vi "Query Capabilities (Aperture).vi"(0 "VISA resource name":refnum<visa-resource-name>, 5 "Absolute Maximums (T)":bool=TRUE, 11 "error in (no error)":errorcluster) -> (4 "VISA resource name out":refnum<visa-resource-name>, 6 "Aperture Min (s)":dbl, 8 "Aperture Max (s)":dbl, 15 "error out":errorcluster)   [LabVIEW 2012, in "NH Research Regenerative Test Series.lvlib"]
doc: "Returns the aperture capabilities of the module in seconds."
uses:
  <instrlib>/NH Research Regenerative Test Series/NH Research Regenerative Test Series.lvlib
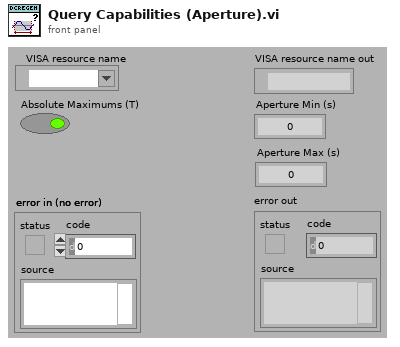
[diagram p1: front panel]
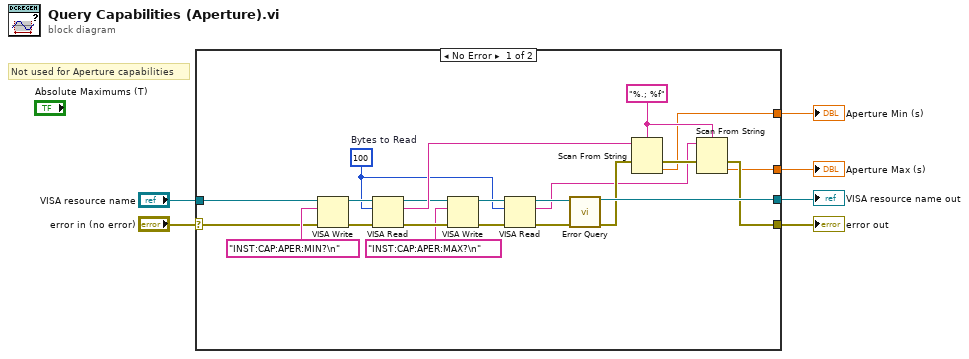
[diagram p0: block diagram]
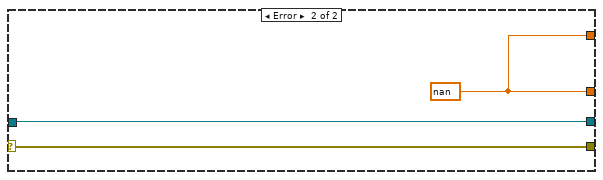
[diagram p2: hidden frame]
diagram:
  # "Not used for Aperture capabilities"
  n1 = case shown="No Error" "error in (no error)" {
    selector: "error in (no error)" -> [w25 w31]
    tunnel: [w10 w31] -> w5
    tunnel: [w22 w30] -> w3
    tunnel: "VISA resource name" -> [w24 w30]
    tunnel: [w9 w29] -> w2
    tunnel: [w8 w29] -> w1
    frame No Error {
      w11 = "%.; %f" ("format string")
      w13 = u32 100  # Bytes to Read
      n2 = VISA Write(VISA resource name=w24, write buffer="INST:CAP:APER:MIN?\n", error in (no error)=w25) -> (VISA resource name out=w27:refnum<visa-resource-name>, error out=w28:errorcluster)  [unwired: 1 out]
      n3 = VISA Read(VISA resource name=w27, byte count=w13, error in (no error)=w28) -> (VISA resource name out=w14:refnum<visa-resource-name>, read buffer=w23:string, error out=w18:errorcluster)  [unwired: 1 out]
      n4 = VISA Write(VISA resource name=w14, write buffer="INST:CAP:APER:MAX?\n", error in (no error)=w18) -> (VISA resource name out=w20:refnum<visa-resource-name>, error out=w19:errorcluster)  [unwired: 1 out]
      n5 = VISA Read(VISA resource name=w20, byte count=w13, error in (no error)=w19) -> (VISA resource name out=w16:refnum<visa-resource-name>, read buffer=w7:string, error out=w17:errorcluster)  [unwired: 1 out]
      n6 = call <instrlib>:"Error Query.vi"("VISA resource name"=w16, "error in (no error)"=w17) -> ("VISA resource name out"=w22:refnum<visa-resource-name>, "error out"=w21:errorcluster)  [unwired: 10 in, 2 out]
      n7 = Scan From String(format string=w11, input string=w23, error in=w21) -> (error out=w12:errorcluster, output 1=w9:dbl)  [unwired: 2 in, 2 out]
      n8 = Scan From String(format string=w11, input string=w7, error in=w12) -> (error out=w10:errorcluster, output 1=w8:dbl)  [unwired: 2 in, 2 out]
    }
    frame Error {
      w29 = nan
    }
  }
  "error out" <- w5
  "VISA resource name out" <- w3
  "Aperture Min (s)" <- w2
  "Aperture Max (s)" <- w1
